vi "InitSolenoids.vi"(8 "error in (no error)":errorcluster) -> (0 "error out":errorcluster, 3 "Array":T1[](array[typedef]))   [LabVIEW 2015]
uses:
  <vilib>/Rock Robotics/WPI/Solenoid/WPI_SolenoidDevRef.ctl
  <vilib>/Rock Robotics/WPI/Solenoid/WPI_SolenoidChannel.ctl
  Framework/Robot Global Data.vi
  <vilib>/Rock Robotics/WPI/Solenoid/WPI_SolenoidOpenSingle.vi
panel:
  in  "Array 2":T1[](array[typedef])
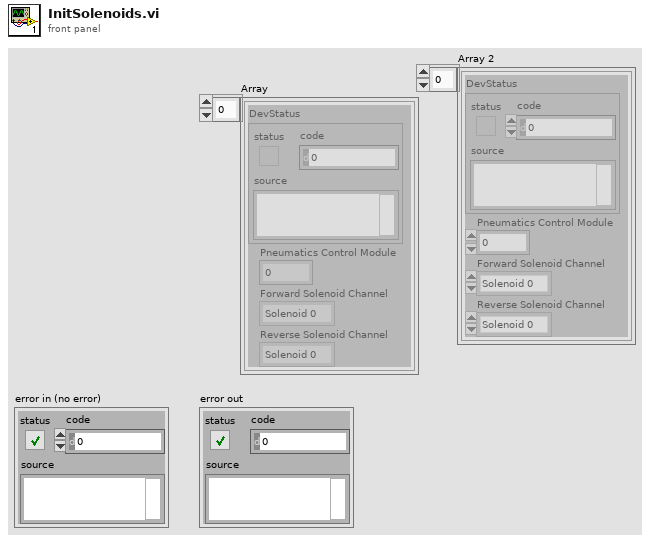
[diagram p1: front panel]
types:
  T1 = typedef "WPI_SolenoidDevRef.ctl" = cluster{"DevStatus":errorcluster, "Pneumatics Control Module":u8, "Forward Solenoid Channel":T2, "Reverse Solenoid Channel":T2}
  T2 = typedef "WPI_SolenoidChannel.ctl" = enum8{"Solenoid 0", "Solenoid 1", "Solenoid 2", "Solenoid 3", "Solenoid 4", "Solenoid 5", "Solenoid 6", "Solenoid 7", "Invalid"}
  T3 = typedef "Robot Type Def.ctl" = enum32{"Disabled", "Ghost", "Casper", "Lofty", "Board", "RaceRobot"}
  T4 = typedef "WPI_CompressorDevRef.ctl" = cluster{"DevStatus":errorcluster, "Pneumatics Control Module":u8}
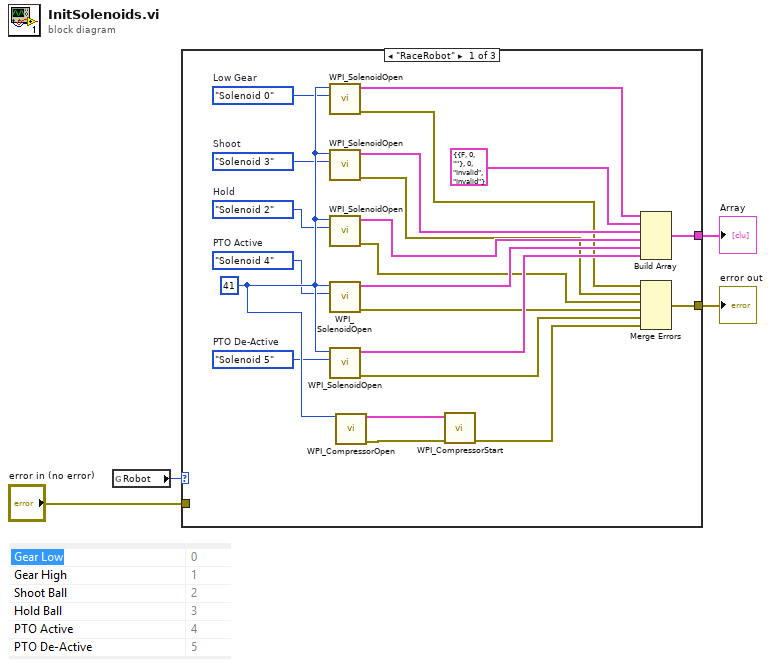
[diagram p0: block diagram]
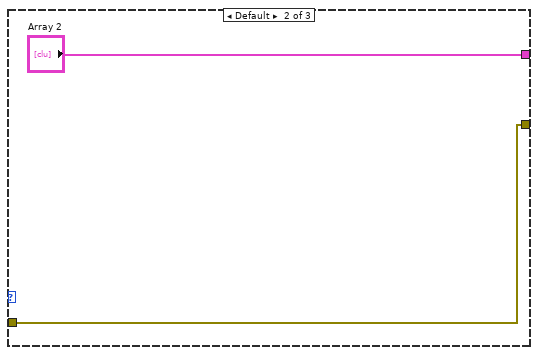
[diagram p2: hidden frame]
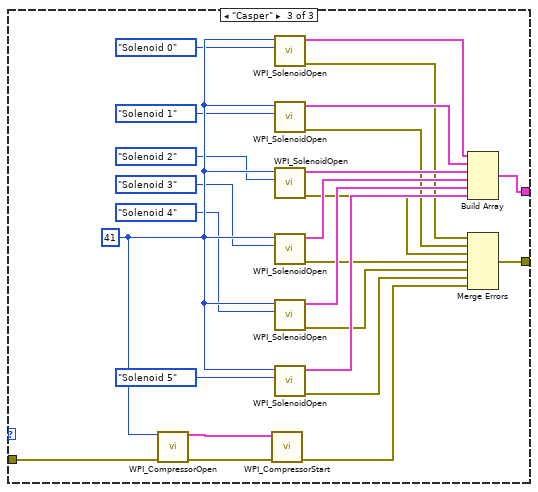
[diagram p3: hidden frame]
diagram:
  n1 = global read "Robot Global Data.vi" "Robot"() -> (w1:T3)
  n2 = case shown="\"RaceRobot\"" w1 {
    tunnel: [w8 "Array 2" w53] -> w4
    tunnel: "error in (no error)" -> [_ w27 w52]
    tunnel: [w7 w27 w38] -> w2
    frame "RaceRobot" {
      w14 = WPI_SolenoidChannel."Solenoid 5"  # PTO De-Active
      w13 = WPI_SolenoidChannel."Solenoid 4"  # PTO Active
      w12 = WPI_SolenoidChannel."Solenoid 2"  # Hold
      w11 = WPI_SolenoidChannel."Solenoid 3"  # Shoot
      w10 = WPI_SolenoidChannel."Solenoid 0"  # Low Gear
      w15 = u8 41 ("Pneumatics Control Module (0)")
      n3 = call-poly <vilib>:"WPI_SolenoidOpen.vi"("Solenoid Channel"=w10, "Pneumatics Control Module (0)"=w15) -> ("error out"=w6:errorcluster, "SolenoidDevRef"=w22:T1)  [unwired: 8 in]
      n4 = call-poly <vilib>:"WPI_SolenoidOpen.vi"("Solenoid Channel"=w11, "Pneumatics Control Module (0)"=w15) -> ("error out"=w17:errorcluster, "SolenoidDevRef"=w23:T1)  [unwired: 8 in]
      n5 = call-poly <vilib>:"WPI_SolenoidOpen.vi"("Solenoid Channel"=w12, "Pneumatics Control Module (0)"=w15) -> ("error out"=w18:errorcluster, "SolenoidDevRef"=w24:T1)  [unwired: 8 in]
      n6 = call-poly <vilib>:"WPI_SolenoidOpen.vi"("Solenoid Channel"=w13, "Pneumatics Control Module (0)"=w15) -> ("error out"=w19:errorcluster, "SolenoidDevRef"=w25:T1)  [unwired: 8 in]
      n7 = call-poly <vilib>:"WPI_SolenoidOpen.vi"("Solenoid Channel"=w14, "Pneumatics Control Module (0)"=w15) -> ("error out"=w20:errorcluster, "SolenoidDevRef"=w26:T1)  [unwired: 8 in]
      n8 = call <vilib>:"WPI_CompressorOpen.vi"("Pneumatics Control Module (0)"=w15) -> ("CompressorDevRef"=w9:T4, "error out"=w16:errorcluster)  [unwired: 13 in]
      n9 = call <vilib>:"WPI_CompressorStart.vi"("error in (no error)"=w16, "CompressorDevRef"=w9) -> ("error out"=w21:errorcluster)  [unwired: 8 in, 1 out]
      n10 = Build Array(w22, T1 {"DevStatus"={"status"=FALSE, "code"=0, "source"=""}, "Pneumatics Control Module"=0, "Forward Solenoid Channel"=enum."Invalid", "Reverse Solenoid Channel"=enum."Invalid"} ("element"), w23, w24, w25, w26) -> (w8:T1[])
      n11 = Merge Errors(w6, w17, w18, w19, w20, w21) -> (w7:errorcluster)
    }
    frame Default {
    }
    frame "Casper" {
      w36 = u8 41 ("Pneumatics Control Module (0)")
      n12 = call <vilib>:"WPI_CompressorOpen.vi"("Pneumatics Control Module (0)"=w36, "error in (no error)"=w52) -> ("CompressorDevRef"=w29:T4, "error out"=w37:errorcluster)  [unwired: 12 in]
      n13 = call <vilib>:"WPI_CompressorStart.vi"("error in (no error)"=w37, "CompressorDevRef"=w29) -> ("error out"=w45:errorcluster)  [unwired: 8 in, 1 out]
      n14 = call-poly <vilib>:"WPI_SolenoidOpen.vi"("Solenoid Channel"=WPI_SolenoidChannel."Solenoid 0", "Pneumatics Control Module (0)"=w36) -> ("error out"=w39:errorcluster, "SolenoidDevRef"=w46:T1)  [unwired: 8 in]
      n15 = call-poly <vilib>:"WPI_SolenoidOpen.vi"("Solenoid Channel"=WPI_SolenoidChannel."Solenoid 1", "Pneumatics Control Module (0)"=w36) -> ("error out"=w40:errorcluster, "SolenoidDevRef"=w47:T1)  [unwired: 8 in]
      n16 = call-poly <vilib>:"WPI_SolenoidOpen.vi"("Solenoid Channel"=WPI_SolenoidChannel."Solenoid 2", "Pneumatics Control Module (0)"=w36) -> ("error out"=w41:errorcluster, "SolenoidDevRef"=w48:T1)  [unwired: 8 in]
      n17 = call-poly <vilib>:"WPI_SolenoidOpen.vi"("Solenoid Channel"=WPI_SolenoidChannel."Solenoid 3", "Pneumatics Control Module (0)"=w36) -> ("error out"=w42:errorcluster, "SolenoidDevRef"=w49:T1)  [unwired: 8 in]
      n18 = call-poly <vilib>:"WPI_SolenoidOpen.vi"("Solenoid Channel"=WPI_SolenoidChannel."Solenoid 4", "Pneumatics Control Module (0)"=w36) -> ("error out"=w43:errorcluster, "SolenoidDevRef"=w50:T1)  [unwired: 8 in]
      n19 = call-poly <vilib>:"WPI_SolenoidOpen.vi"("Solenoid Channel"=WPI_SolenoidChannel."Solenoid 5", "Pneumatics Control Module (0)"=w36) -> ("error out"=w44:errorcluster, "SolenoidDevRef"=w51:T1)  [unwired: 8 in]
      n20 = Build Array(w46, w47, w48, w49, w50, w51) -> (w53:T1[])
      n21 = Merge Errors(w39, w40, w41, w42, w43, w44, w45) -> (w38:errorcluster)
    }
  }
  "Array" <- w4
  "error out" <- w2
